vi "init.vi"(8 "error in (no error)":errorcluster, 11 "DAQ  in":refnum<class "DAQ .lvclass">) -> (0 "error out":errorcluster, 3 "DAQ  out":refnum<class "DAQ .lvclass">)   [LabVIEW 2026, in "Hardware.lvlib" / "DAQ .lvclass"]
uses:
  DAQ .lvclass
  MAL-Framework/user.lib/Common Components/Hardware/Hardware.lvclass
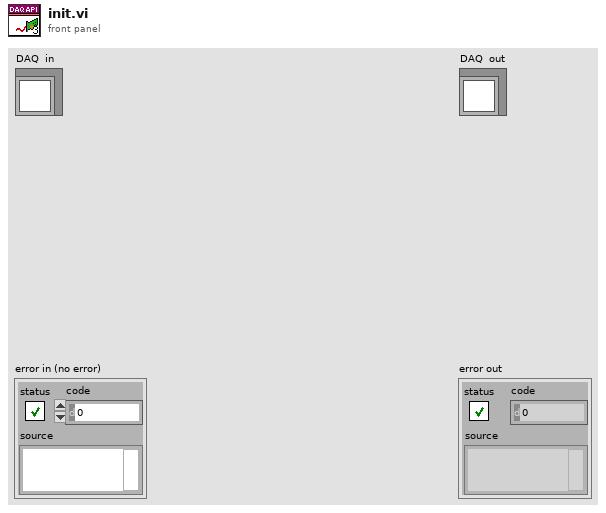
[diagram p1: front panel]
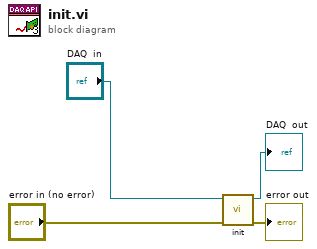
[diagram p0: block diagram]
diagram:
  n1 = call-parent "init.vi"("error in (no error)"="error in (no error)", "Hardware in"="DAQ  in") -> ("error out"=→"error out":errorcluster, "Hardware out"=→"DAQ  out":refnum<class "DAQ .lvclass">)  [unwired: 8 in]
